vi "读取MB session in.vi"(8 "error in (no error)":errorcluster caption="错误输入（无错误）", 11 "HL7输入":refnum<class "HL7.lvclass">) -> (0 "error out":errorcluster caption="错误输出", 2 "MB Serial Master:MB_Master":refnum<class "MB_Master.lvclass">, 3 "HL7输出":refnum<class "HL7.lvclass">)   [LabVIEW 2016, in "HL7.lvlib" / "HL7.lvclass"]
uses:
  HL7.lvclass
  <vilib>/Plasmionique/MB Master/MB_Master/MB_Master.lvclass
  HL7.lvclass/HL7.ctl
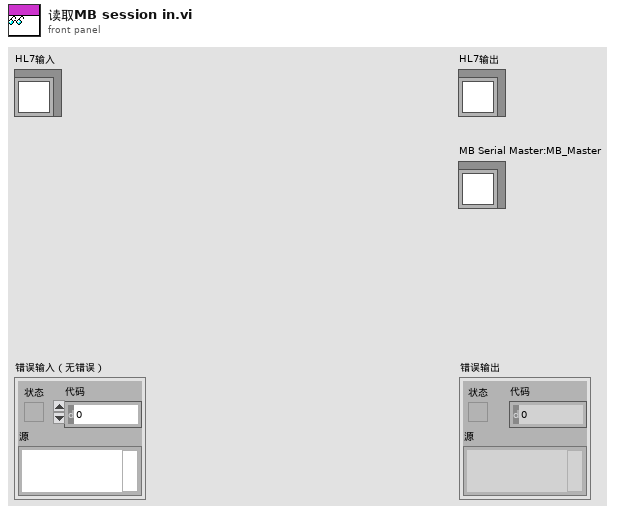
[diagram p1: front panel]
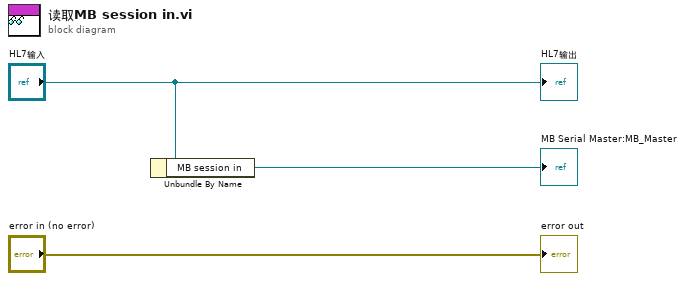
[diagram p0: block diagram]
diagram:
  n1 = Unbundle By Name("HL7输入") -> ("MB session in"=→"MB Serial Master:MB_Master":refnum<class "MB_Master.lvclass">)
  "error out" <- "error in (no error)"
  "HL7输出" <- "HL7输入"
